vi "Display Info.vi"(7 "Layout ref":refnum<vi>, 8 "error in (no error)":errorcluster, 9 "Modify (F) /Add [T]":bool, 10 "Names in use":string[](array[string]), 11 "TestMenu in":refnum<class "TestMenu.lvclass">) -> (0 "error out":errorcluster, 1 "Names in use out":string[](array[string]), 2 "Changes Made?":bool, 3 "TestMenu out":refnum<class "TestMenu.lvclass">)   [LabVIEW 2013, in "TestMenu.lvclass"]
uses:
  TestMenu.lvclass
  Device/Device.lvclass
panel:
  # "This VI just sets the wiring structure.\nOpen a child override version instead!"
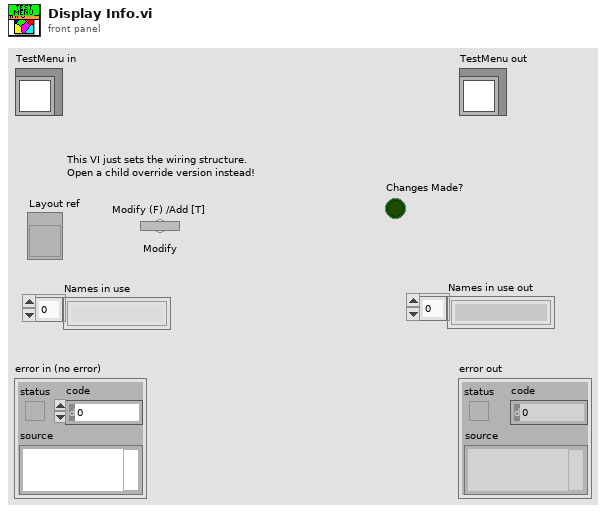
[diagram p1: front panel]
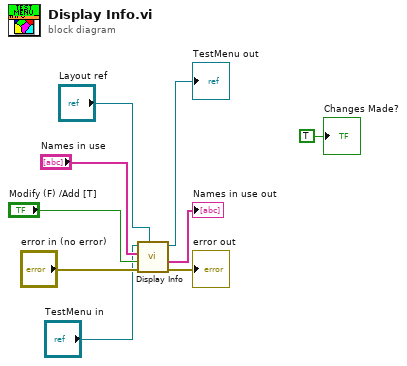
[diagram p0: block diagram]
diagram:
  n1 = call-parent "Display Info.vi"("Layout ref"="Layout ref", "error in (no error)"="error in (no error)", "Modify (F) /Add [T]"="Modify (F) /Add [T]", "Names in use"="Names in use", "Device in"="TestMenu in") -> ("error out"=→"error out":errorcluster, "Names in use out"=→"Names in use out":string[], "Device out"=→"TestMenu out":refnum<class "TestMenu.lvclass">)  [unwired: 3 in, 1 out]
  "Changes Made?" <- TRUE ("Changes Made?")
